vi "LIA.GetMagnitude.vi"(8 "error in (no error)":errorcluster, 11 "LIA.SR810 in":refnum<class "LIA.SR810.lvclass">) -> (0 "error out":errorcluster, 2 "Magnitude":dbl, 3 "LIA.SR810 out":refnum<class "LIA.SR810.lvclass">)   [LabVIEW 2017, in "LIA.SR810.lvclass"]
uses:
  LIA.SR810.lvclass
  <instrlib>/Stanford Research 830/Public/Data/Read (1 Parameter).vi
  <instrlib>/Stanford Research 830/Stanford Research 830.lvlib
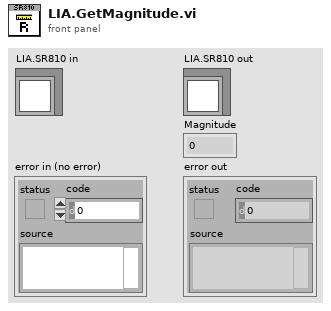
[diagram p1: front panel]
types:
  T1 = cluster{"VISA resource":refnum<visa-resource-name>}
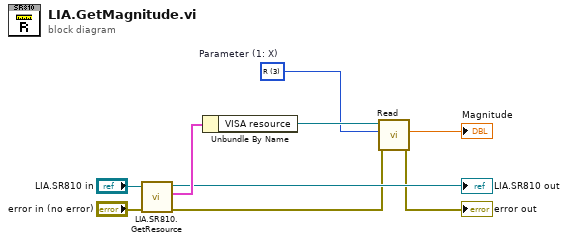
[diagram p0: block diagram]
diagram:
  w4 = u16 3 items=["X"=1, "Y"=2, "R"=3, "Theta"=4, "Channel 1"=5, "Channel 2"=6, "Aux In 1"=7, "Aux In 2"=8, "Aux In 3"=9, "Aux In 4"=10]  # Parameter (1: X)
  n1 = call "LIA.SR810.GetResource.vi"("error in (no error)"="error in (no error)", "LIA.SR810 in"="LIA.SR810 in") -> ("error out"=w3:errorcluster, "Resource"=w7:T1, "LIA.SR810 out"=→"LIA.SR810 out":refnum<class "LIA.SR810.lvclass">)  [unwired: 7 in]
  n2 = Unbundle By Name(w7) -> ("VISA resource"=w5:refnum<visa-resource-name>)
  n3 = call-poly <instrlib>:"Read.vi"("error in (no error)"=w3, "Parameter (1: X)"=w4, "VISA resource name"=w5) -> ("error out"=→"error out":errorcluster, "Measurement"=→"Magnitude":dbl)  [unwired: 6 in, 1 out]
